vi "Poly_ReadStepper.vi"   [LabVIEW 2012]
doc: "Reads the stepper wired to the specified \"Port\" and returns the read value as \"Variable Out\"."
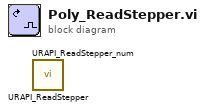
[diagram p0: block diagram]
diagram:
  n1 = call <userlib>:"URAPI_ReadStepper.vi"() -> ()  [unwired: 4 in, 2 out]
  n2 = call <userlib>:"URAPI_ReadStepper_num.vi"() -> ()  [unwired: 4 in, 2 out]
